vi "fgv_prechirper set values.vi"(7 "FGV Actions":T1, 8 "error in (no error)":errorcluster, 10 "Prism A value [IN]":i32, 11 "Prism B value [IN]":i32) -> (0 "error out":errorcluster, 2 "Prism B value [OUT]":i32, 3 "Prism A value [OUT]":i32)   [LabVIEW 2017]
uses:
  Typedefs/fgv_actions.ctl
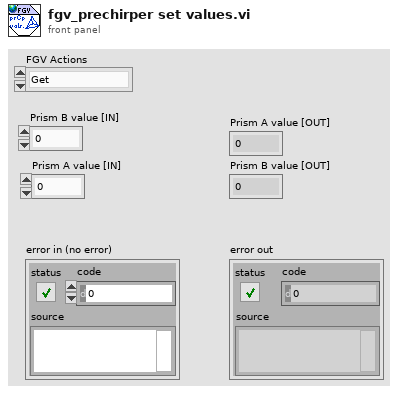
[diagram p1: front panel]
types:
  T1 = typedef "fgv_actions.ctl" = enum16{"Get", "Set"}
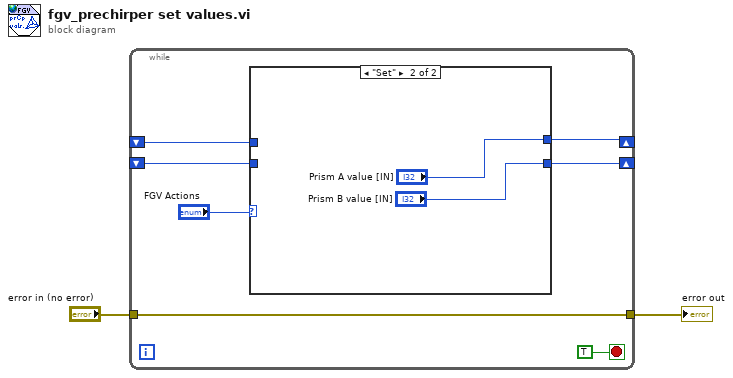
[diagram p0: block diagram]
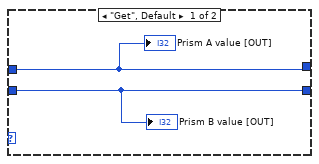
[diagram p2: hidden frame]
diagram:
  n1 = while {
    shift-right: [w7] -> _
    shift-left: _ -> [w6]
    shift-right: [w5] -> _
    shift-left: _ -> [w4]
    tunnel: "error in (no error)" -> [w3]
    tunnel: [w3] -> w1
    stop <- TRUE stop-if-true
    n2 = case shown="\"Set\"" "FGV Actions" {
      tunnel: [w11 "Prism A value [IN]"] -> w7
      tunnel: w6 -> [w11 _]
      tunnel: [w10 "Prism B value [IN]"] -> w5
      tunnel: w4 -> [w10 _]
      frame "Get", Default {
        "Prism A value [OUT]" <- w11
        "Prism B value [OUT]" <- w10
      }
      frame "Set" {
      }
    }
  }
  "error out" <- w1
